vi "Process Mouse Move.vi"(10 "Coords":T5, 11 "Core Data in":T1) -> (3 "Core Data out":T1)   [LabVIEW 2022 SP3, in "Application.lvlib"]
uses:
  Application.lvlib
  <vilib>/Utility/miscctls.llb/LVPoint32TypeDef.ctl
  Core Data.ctl
  Scene/Scene.lvclass
  Libraries/3D/Transform.ctl
  Libraries/3D/Vector 3D.ctl
  Mouse Button Held.ctl
  Libraries/3D/3D.lvlib
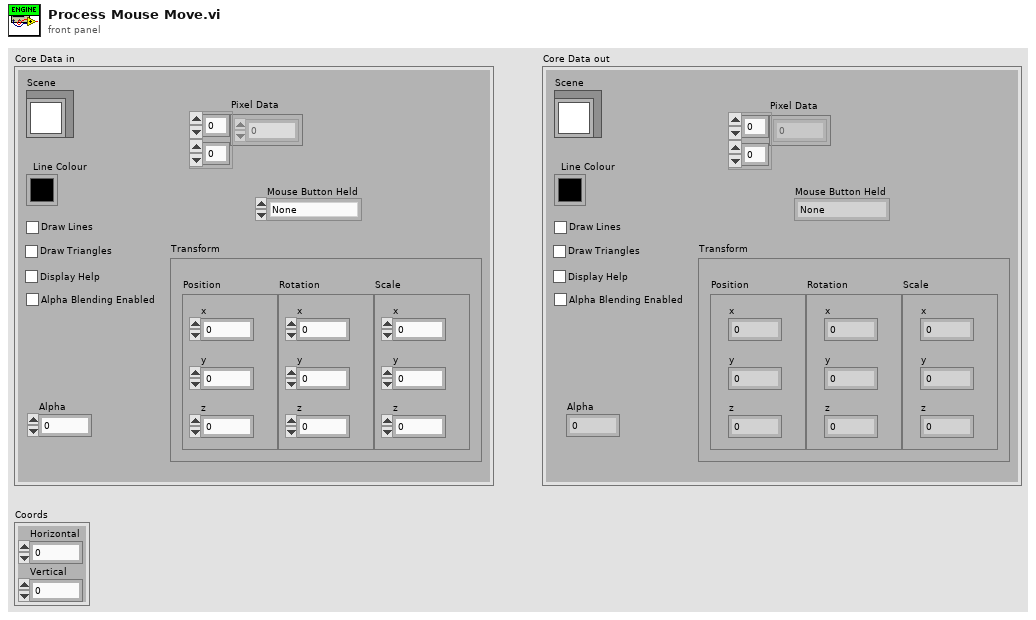
[diagram p1: front panel]
types:
  T1 = typedef "Application.lvlib/Core Data.ctl" = cluster{"Line Colour":u32, "Draw Lines":bool, "Draw Triangles":bool, "Pixel Data":u32[][], "Scene":refnum<class "Scene.lvclass">, "Display Help":bool, "Transform":T2, "Alpha":dbl, "Mouse Button Held":T4, "Alpha Blending Enabled":bool}
  T2 = typedef "3D.lvlib/Transform.ctl" = cluster{"Position":T3, "Rotation":T3, "Scale":T3}
  T3 = typedef "3D.lvlib/Vector 3D.ctl" = cluster{"x":sgl, "y":sgl, "z":sgl}
  T4 = typedef "Application.lvlib/Mouse Button Held.ctl" = enum16{"None", "Left", "Middle", "Right"}
  T5 = typedef "LVPoint32TypeDef.ctl" = cluster{"Horizontal":i32, "Vertical":i32}
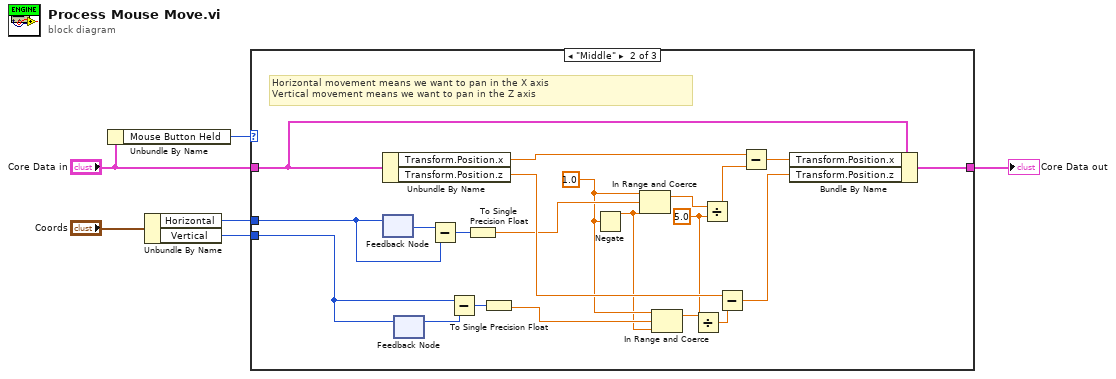
[diagram p0: block diagram]
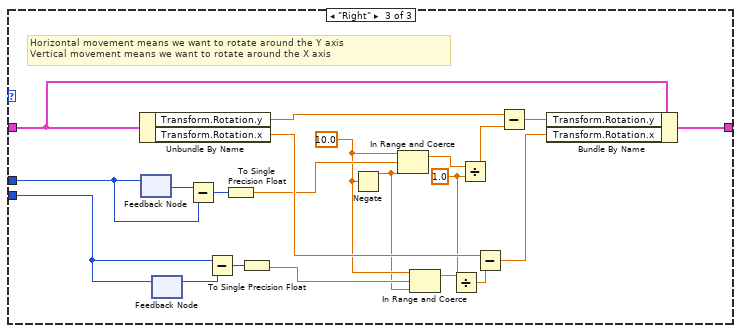
[diagram p3: hidden frame]
diagram:
  n1 = Unbundle By Name("Core Data in") -> ("Mouse Button Held"=w3:T4)
  n2 = Unbundle By Name("Coords") -> ("Horizontal"=w2:i32, "Vertical"=w1:i32)
  n3 = case shown="\"Middle\"" w3 {
    tunnel: [w7 w28 w49] -> w5
    tunnel: w2 -> [_ w25 w46]
    tunnel: "Core Data in" -> [w7 w20 w41]
    tunnel: w1 -> [_ w17 w38]
    frame "None", Default {
    }
    frame "Middle" {
      w8 = sgl 5.0 ("y")
      w14 = sgl 1.0 ("upper limit")
      # "Horizontal movement means we want to pan in the X axis\nVertical movement means we want to pan in the Z axis"
      n4 = Unbundle By Name(w20) -> ("Transform.Position.x"=w27:sgl, "Transform.Position.z"=w22:sgl)
      n5 = feedback #1() -> (w24:i32)  [unwired: 1 in]
      n6 = feedback-in #1(w25) -> ()
      n7 = feedback #2() -> (w23:i32)  [unwired: 1 in]
      n8 = feedback-in #2(w17) -> ()
      n9 = Subtract(x=w24, y=w25) -> (x-y=w19:i32)
      n10 = Subtract(x=w17, y=w23) -> (x-y=w18:i32)
      n11 = To Single Precision Float(number=w19) -> (single precision float=w16:sgl)
      n12 = To Single Precision Float(number=w18) -> (single precision float=w15:sgl)
      n13 = Negate(x=w14) -> (-x=w13:sgl)
      n14 = In Range and Coerce(upper limit=w14, x=w16, lower limit=w13) -> (coerced(x)=w12:sgl)  [unwired: 1 out]
      n15 = In Range and Coerce(upper limit=w14, x=w15, lower limit=w13) -> (coerced(x)=w10:sgl)  [unwired: 1 out]
      n16 = Divide(x=w10, y=w8) -> (x/y=w9:sgl)
      n17 = Divide(x=w12, y=w8) -> (x/y=w11:sgl)
      n18 = Subtract(x=w22, y=w9) -> (x-y=w21:sgl)
      n19 = Subtract(x=w27, y=w11) -> (x-y=w26:sgl)
      n20 = Bundle By Name(cluster=w20, "Transform.Position.x"=w26, "Transform.Position.z"=w21) -> (w28:T1)
    }
    frame "Right" {
      w29 = sgl 1.0 ("y")
      w35 = sgl 10.0 ("upper limit")
      # "Horizontal movement means we want to rotate around the Y axis\nVertical movement means we want to rotate around the X axis"
      n21 = Unbundle By Name(w41) -> ("Transform.Rotation.y"=w48:sgl, "Transform.Rotation.x"=w43:sgl)
      n22 = feedback #3() -> (w45:i32)  [unwired: 1 in]
      n23 = feedback-in #3(w46) -> ()
      n24 = feedback #4() -> (w44:i32)  [unwired: 1 in]
      n25 = feedback-in #4(w38) -> ()
      n26 = Subtract(x=w45, y=w46) -> (x-y=w40:i32)
      n27 = Subtract(x=w38, y=w44) -> (x-y=w39:i32)
      n28 = To Single Precision Float(number=w40) -> (single precision float=w37:sgl)
      n29 = To Single Precision Float(number=w39) -> (single precision float=w36:sgl)
      n30 = Negate(x=w35) -> (-x=w34:sgl)
      n31 = In Range and Coerce(upper limit=w35, x=w37, lower limit=w34) -> (coerced(x)=w33:sgl)  [unwired: 1 out]
      n32 = In Range and Coerce(upper limit=w35, x=w36, lower limit=w34) -> (coerced(x)=w31:sgl)  [unwired: 1 out]
      n33 = Divide(x=w31, y=w29) -> (x/y=w30:sgl)
      n34 = Divide(x=w33, y=w29) -> (x/y=w32:sgl)
      n35 = Subtract(x=w43, y=w30) -> (x-y=w42:sgl)
      n36 = Subtract(x=w48, y=w32) -> (x-y=w47:sgl)
      n37 = Bundle By Name(cluster=w41, "Transform.Rotation.y"=w47, "Transform.Rotation.x"=w42) -> (w49:T1)
    }
  }
  "Core Data out" <- w5
